vi "distance.vi"() -> ()   [LabVIEW 2015]
panel:
  in  "camra distance":dbl
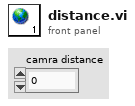
[diagram p1: front panel]
diagram:
